vi "Flow Out AFM.vi"() -> ()   [LabVIEW 2017]
panel:
  out "Flow Out":dbl
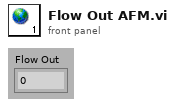
[diagram p1: front panel]
diagram:
